vi "Create Field.vi"(1 "RelGraphSize":sgl=1.2, 2 "LineIntensity":dbl=100.0) -> (0 "Intensity Graph":dbl[][](graph))   [LabVIEW 2014, in "Field.lvclass"]
uses:
  Field.lvclass
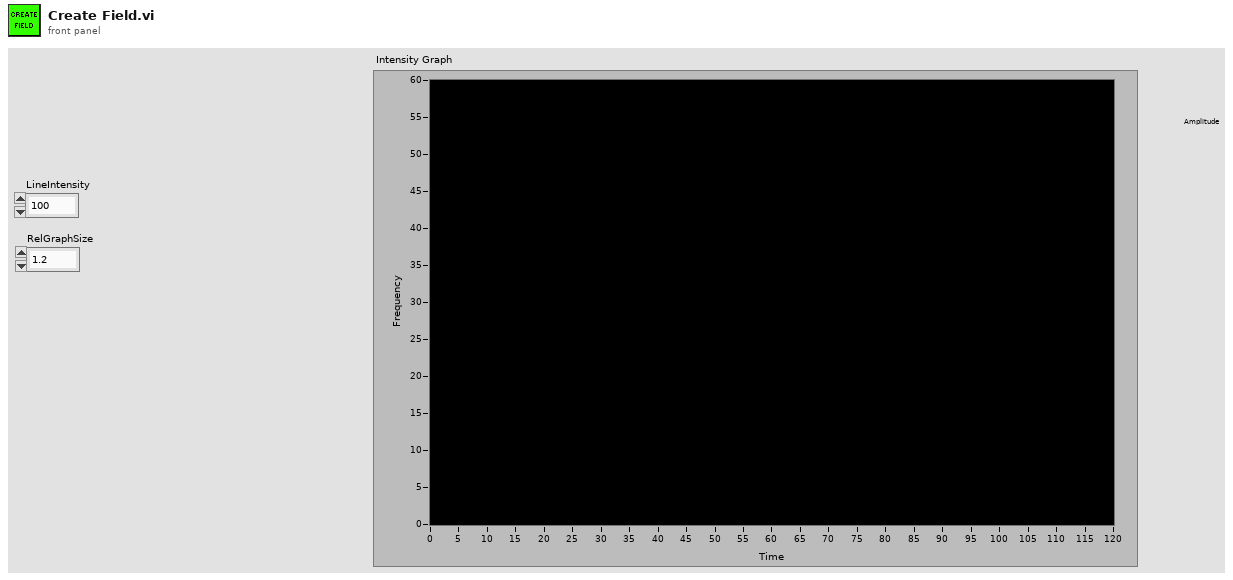
[diagram p1: front panel]
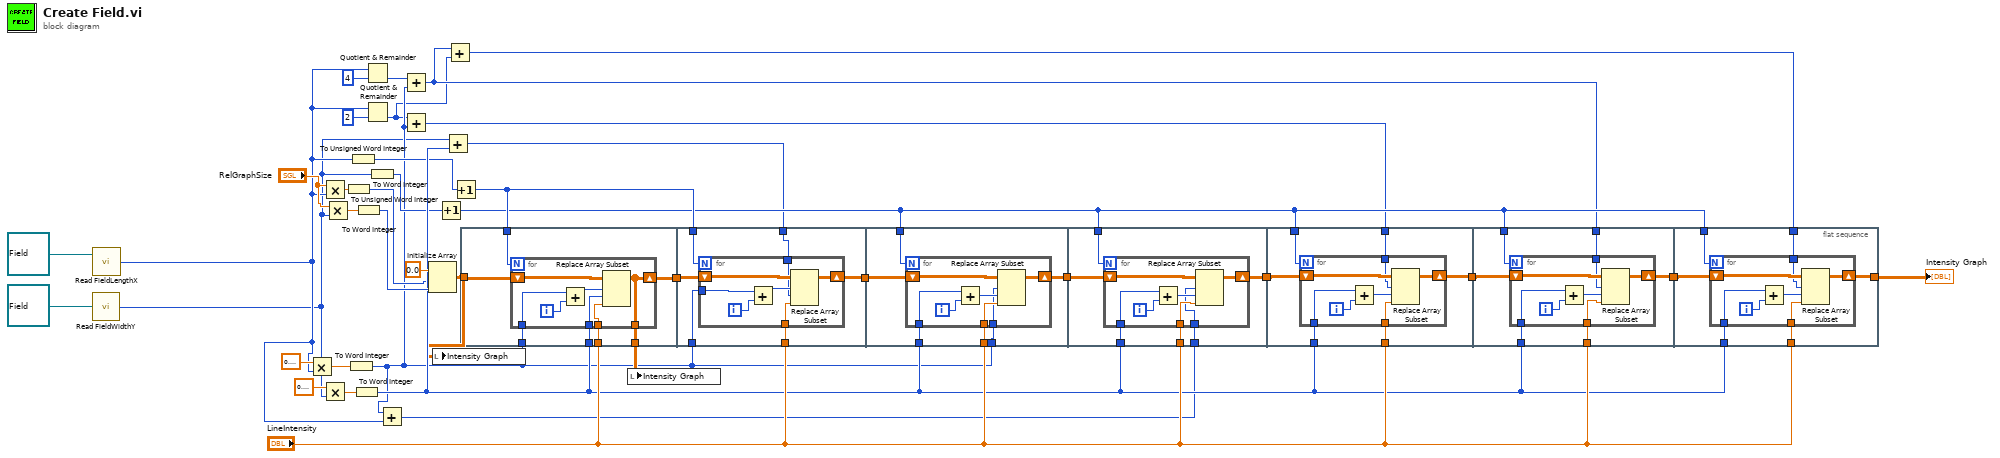
[diagram p0: block diagram]
diagram:
  n1 = call-dynamic "Read FieldWidthY.vi"("Field in"=refnum<class "Field.lvclass"> refnum) -> ("FieldWidthY"=w3:i32)  [unwired: 1 in, 2 out]
  n2 = call-dynamic "Read FieldLengthX.vi"("Field in"=refnum<class "Field.lvclass"> refnum) -> ("FieldLengthX"=w4:i32)  [unwired: 1 in, 2 out]
  n3 = Multiply(x=sgl 0.1 ("FieldLengthX"), y=w4) -> (x*y=w23:sgl)
  n4 = Multiply(x="RelGraphSize", y=w4) -> (x*y=w29:sgl)
  n5 = Multiply(x=sgl 0.1 ("FieldLengthX"), y=w3) -> (x*y=w21:sgl)
  n6 = Multiply(x="RelGraphSize", y=w3) -> (x*y=w30:sgl)
  n7 = To Unsigned Word Integer(number=w29) -> (unsigned 16bit integer=w15:u16)
  n8 = To Word Integer(number=w23) -> (16bit integer=w7:i16)
  n9 = To Unsigned Word Integer(number=w4) -> (unsigned 16bit integer=w14:u16)
  n10 = To Word Integer(number=w21) -> (16bit integer=w20:i16)
  n11 = To Word Integer(number=w30) -> (16bit integer=w27:i16)
  n12 = Quotient & Remainder(x=w4, y=u8 4) -> (floor(x/y)=w9:i32)  [unwired: 1 out]
  n13 = Quotient & Remainder(x=w4, y=u8 2) -> (floor(x/y)=w5:i32)  [unwired: 1 out]
  n14 = To Word Integer(number=w3) -> (16bit integer=w13:i16)
  n15 = Add(x=w7, y=w4) -> (x+y=w12:i32)
  n16 = Add(x=w9, y=w7) -> (x+y=w8:i32)
  n17 = Add(x=w5, y=w7) -> (x+y=w11:i32)
  n18 = Initialize Array(0.0 ("element"), w15, w27) -> (w17:dbl[][])
  n19 = local write "Intensity Graph"(w17) -> ()
  n20 = Increment(x=w13) -> (x+1=w26:i16)
  n21 = Add(x=w3, y=w20) -> (x+y=w18:i32)
  n22 = Add(x=w8, y=w5) -> (x+y=w6:i32)
  n23 = Increment(x=w14) -> (x+1=w28:u16)
  n24 = flat-sequence {
    tunnel: w17 -> [w46]
    tunnel: [w45] -> w39
    tunnel: w28 -> [w44]
    tunnel: w7 -> [w43]
    tunnel: w20 -> [w42]
    tunnel: "LineIntensity" -> [w41]
    tunnel: [w40] -> w16
    tunnel: w39 -> [w59]
    tunnel: [w58] -> w38
    tunnel: w28 -> [w57]
    tunnel: w7 -> [w56]
    tunnel: "LineIntensity" -> [w55]
    tunnel: w18 -> [w54]
    tunnel: w38 -> [w72]
    tunnel: [w71] -> w37
    tunnel: w26 -> [w70]
    tunnel: w20 -> [w69]
    tunnel: "LineIntensity" -> [w68]
    tunnel: w7 -> [w67]
    tunnel: w37 -> [w85]
    tunnel: [w84] -> w36
    tunnel: w26 -> [w83]
    tunnel: w20 -> [w82]
    tunnel: "LineIntensity" -> [w81]
    tunnel: w12 -> [w80]
    tunnel: w36 -> [w97]
    tunnel: [w98] -> w35
    tunnel: w26 -> [w96]
    tunnel: w20 -> [w95]
    tunnel: "LineIntensity" -> [w94]
    tunnel: w11 -> [w93]
    tunnel: w35 -> [w111]
    tunnel: [w110] -> w34
    tunnel: w26 -> [w109]
    tunnel: w20 -> [w108]
    tunnel: "LineIntensity" -> [w107]
    tunnel: w8 -> [w106]
    tunnel: [w123] -> w32
    tunnel: w34 -> [w124]
    tunnel: w26 -> [w122]
    tunnel: w20 -> [w121]
    tunnel: "LineIntensity" -> [w120]
    tunnel: w6 -> [w119]
    frame #0 {
      n25 = for {
        N: w44 -> [_]
        shift-right: [w47] -> w45
        shift-left: w46 -> [w53]
        tunnel: w43 -> [w50]
        tunnel: w42 -> [w49]
        tunnel: w41 -> [w48]
        tunnel: [w47] -> w40
        i -> [w52]
        n26 = Add(x=w50, y=w52) -> (x+y=w51:i32)
        n27 = Replace Array Subset(array=w53, new element=w48, index (row)=w51, index (col)=w49) -> (w47:dbl[][])
      }
    }
    frame #1 {
      n28 = for {
        N: w57 -> [_]
        shift-right: [w63] -> w58
        shift-left: w59 -> [w66]
        tunnel: w56 -> [w62]
        tunnel: w55 -> [w61]
        tunnel: w54 -> [w60]
        i -> [w65]
        n29 = Add(x=w62, y=w65) -> (x+y=w64:i32)
        n30 = Replace Array Subset(array=w66, new element=w61, index (row)=w64, index (col)=w60) -> (w63:dbl[][])
      }
    }
    frame #2 {
      n31 = for {
        N: w70 -> [_]
        shift-right: [w77] -> w71
        shift-left: w72 -> [w79]
        tunnel: w69 -> [w75]
        tunnel: w68 -> [w74]
        tunnel: w67 -> [w73]
        i -> [w78]
        n32 = Add(x=w75, y=w78) -> (x+y=w76:i32)
        n33 = Replace Array Subset(array=w79, new element=w74, index (row)=w73, index (col)=w76) -> (w77:dbl[][])
      }
    }
    frame #3 {
      n34 = for {
        N: w83 -> [_]
        shift-right: [w90] -> w84
        shift-left: w85 -> [w92]
        tunnel: w82 -> [w88]
        tunnel: w81 -> [w87]
        tunnel: w80 -> [w86]
        i -> [w91]
        n35 = Add(x=w88, y=w91) -> (x+y=w89:i32)
        n36 = Replace Array Subset(array=w92, new element=w87, index (row)=w86, index (col)=w89) -> (w90:dbl[][])
      }
    }
    frame #4 {
      n37 = for {
        N: w96 -> [_]
        shift-right: [w103] -> w98
        shift-left: w97 -> [w105]
        tunnel: w95 -> [w101]
        tunnel: w94 -> [w100]
        tunnel: w93 -> [w99]
        i -> [w104]
        n38 = Add(x=w101, y=w104) -> (x+y=w102:i32)
        n39 = Replace Array Subset(array=w105, new element=w100, index (row)=w99, index (col)=w102) -> (w103:dbl[][])
      }
    }
    frame #5 {
      n40 = for {
        N: w109 -> [_]
        shift-right: [w116] -> w110
        shift-left: w111 -> [w118]
        tunnel: w108 -> [w114]
        tunnel: w107 -> [w113]
        tunnel: w106 -> [w112]
        i -> [w117]
        n41 = Add(x=w114, y=w117) -> (x+y=w115:i32)
        n42 = Replace Array Subset(array=w118, new element=w113, index (row)=w112, index (col)=w115) -> (w116:dbl[][])
      }
    }
    frame #6 {
      n43 = for {
        N: w122 -> [_]
        shift-right: [w129] -> w123
        shift-left: w124 -> [w131]
        tunnel: w121 -> [w127]
        tunnel: w120 -> [w126]
        tunnel: w119 -> [w125]
        i -> [w130]
        n44 = Add(x=w127, y=w130) -> (x+y=w128:i32)
        n45 = Replace Array Subset(array=w131, new element=w126, index (row)=w125, index (col)=w128) -> (w129:dbl[][])
      }
    }
  }
  n46 = local write "Intensity Graph"(w16) -> ()
  "Intensity Graph" <- w32
